vi "17.DMA-FIFO.vi"() -> ()   [LabVIEW 2019]
uses:
  <vilib>/rvi/Emulation/niFpgaGetClockAttributes.vi
  <vilib>/rvi/Emulation/niFpgaSctlEmulationGetInTimedLoop.vi
  <vilib>/rvi/Emulation/niFpgaEmulationReportErrorSimple.vi
  <vilib>/rvi/eio/common/nirviEmuTemplateMethod_errors.vi
  <vilib>/rvi/interface/RandomDataEmulation/niFpgaRandomDataHandleErrors.vi
  <vilib>/rvi/Emulation/niFpgaProcessEmulError.vi
  <vilib>/rvi/Emulation/niFpgaCriticalErrorInLSC.vi
  <vilib>/eio/EIONode/EIONode.xnode
  <vilib>/rvi/DataTransferAndStorage/Container/XNode/niFpgaContainer.xnode
  <vilib>/rvi/interface/RandomDataEmulation/nirviRandomDataFpgaReadWriteTemplate.vi
panel:
  out "Overflow?":bool
  in  "DMA Cleared?":bool
  in  "Count(uSec)":u32 caption="计数器(uSec)"
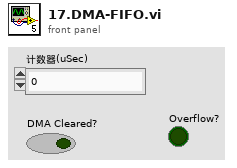
[diagram p1: front panel]
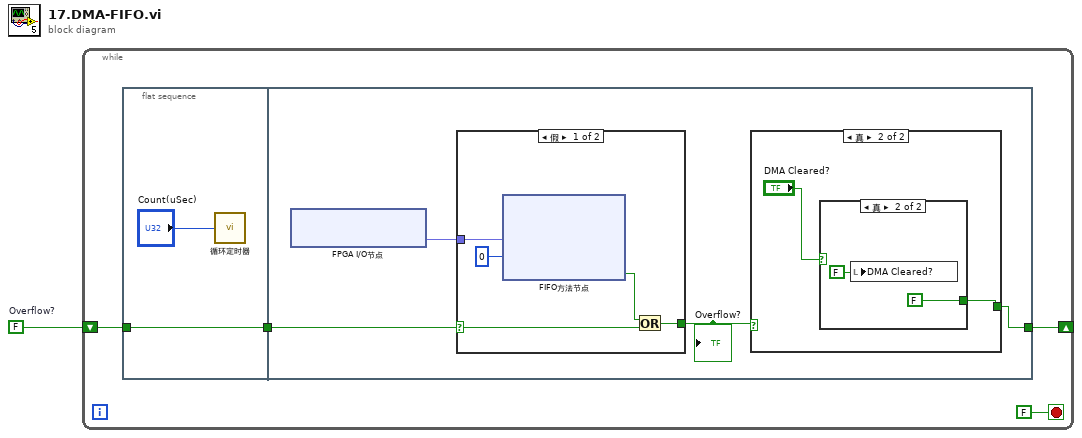
[diagram p0: block diagram]
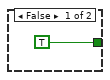
[diagram p3: hidden frame]
diagram:
  w1 = FALSE  # Overflow?
  n1 = while {
    shift-right: [w3] -> _
    shift-left: w1 -> [w5]
    stop <- FALSE stop-if-true
    n2 = flat-sequence {
      tunnel: w5 -> [w6]
      tunnel: [w6] -> w4
      tunnel: w4 -> [w11]
      tunnel: [w8] -> w3
      frame #0 {
        n3 = call "循环定时器"("Count(uSec)"="Count(uSec)") -> ()  [unwired: 1 out]
      }
      frame #1 {
        n4 = xnode "FPGA I/O节点"() -> ("ConnectorB/AI0"=w10:fxp<+/-,24,5>)  [unwired: 1 in, 1 out]
        n5 = case shown="假" w11 {
          selector: w11 -> [w18 w23]
          tunnel: w10 -> [w22 _]
          tunnel: [w20 w23] -> w9
          frame False {
            n6 = xnode ("FIFO方法节点")("元素"=w22, "超时"=0) -> ("超时？"=w19:bool)  [unwired: 1 in, 1 out]
            n7 = Or(x=w19, y=w18) -> (x .or. y?=w20:bool)
          }
          frame True {
          }
        }
        "Overflow?" <- w9
        n8 = case shown="真" w9 {
          selector: w9 -> [w12 _]
          tunnel: [w12 w13] -> w8
          frame False {
          }
          frame True {
            n9 = case shown="真" "DMA Cleared?" {
              tunnel: [TRUE FALSE] -> w13
              frame False {
              }
              frame True {
                n10 = local write "DMA Cleared?"(FALSE) -> ()
              }
            }
          }
        }
      }
    }
  }
